vi "ChannelSounder.vi"() -> ()   [LabVIEW 2018]
uses:
  <instrlib>/niUSRP/niUSRP Fetch Rx Data (CDB WDT).vi
  <vilib>/measure/maspectr.llb/FFT Power Spectrum and PSD for 1 Chan (CDB).vi
  <vilib>/measure/NI_MAPro.lvlib
panel:
  out "Acquired Signal":waveform(dbl)[](graph)
  out "Waveform Graph":cluster{"f0":dbl, "df":dbl, "magnitude":dbl[]}(graph)
  in  "number of samples":i64=100000
  in  "stop":bool
  out "error out":errorcluster
  out "coerced gain":dbl format="%#_6f"
  out "coerced carrier frequency":dbl=100000.0 format="%#_6p"
  out "coerced IQ rate":dbl=100000.0 format="%#_6p"
  in  "active antenna":string="RX2"
  in  "carrier frequency":dbl=867999999.0 format="%#_6p"
  in  "IQ rate":dbl=100000.0 format="%#_6p"
  in  "Rx gain [dB]":dbl format="%#_6f"
  in  "device IP":refnum<k15>="192.168.10.2"
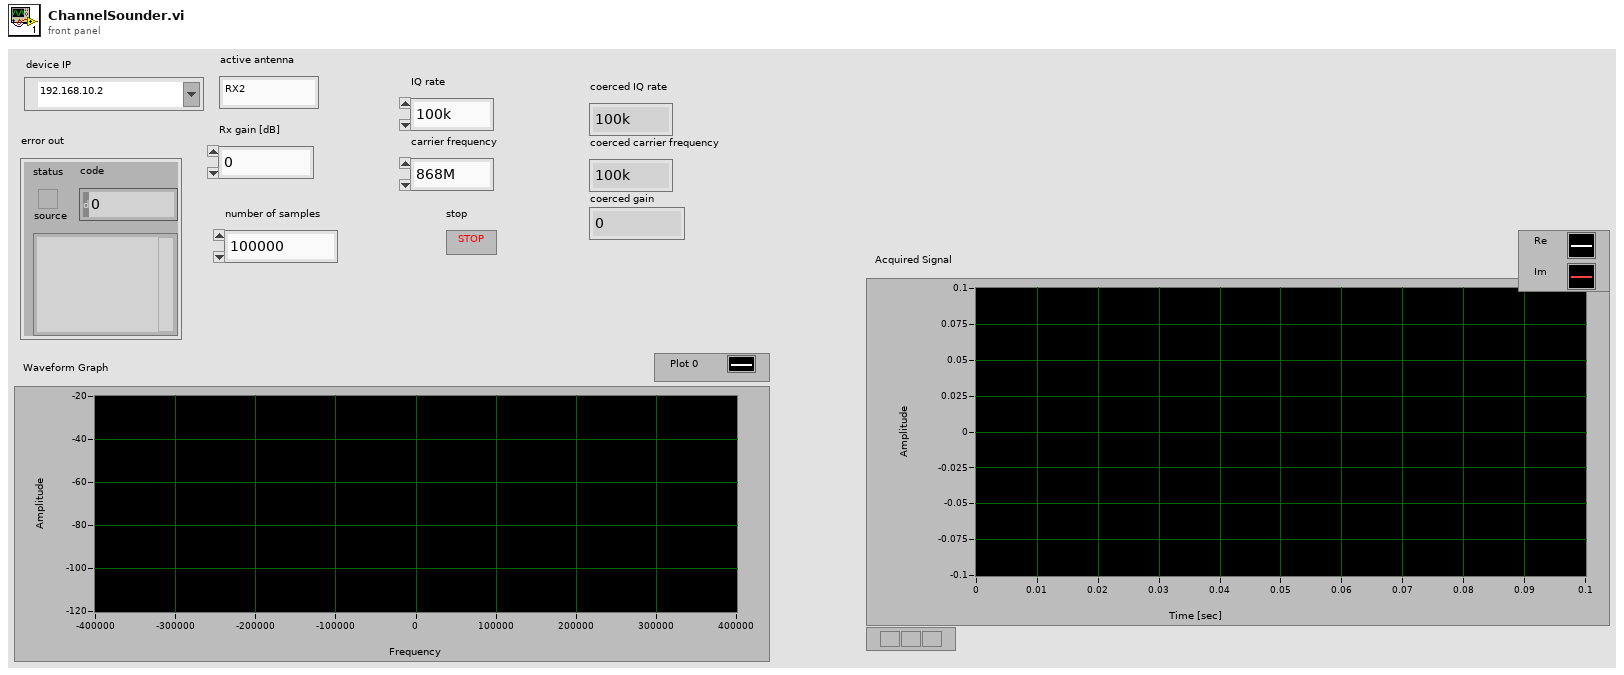
[diagram p1: front panel]
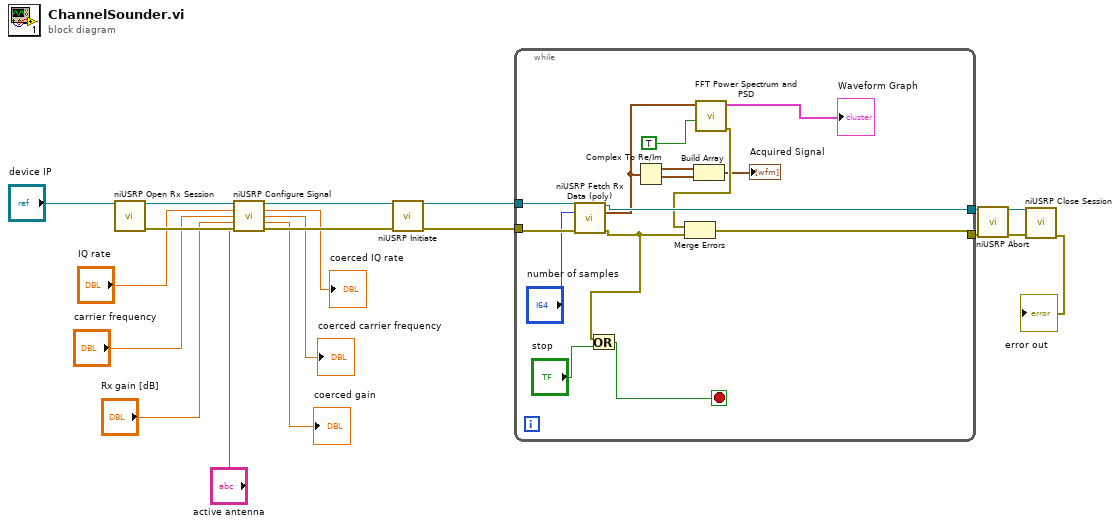
[diagram p0: block diagram]
diagram:
  n1 = call <instrlib>:"niUSRP Open Rx Session.vi"("device names"="device IP") -> ("session handle out"=w19:refnum<k15>, "error out"=w18:errorcluster)  [unwired: 13 in]
  n2 = call <instrlib>:"niUSRP Configure Signal.vi"("session handle"=w19, "IQ rate"="IQ rate", "carrier frequency"="carrier frequency", "gain"="Rx gain [dB]", "error in (no error)"=w18, "active antenna"="active antenna") -> ("session handle out"=w17:refnum<k15>, "coerced IQ rate"=→"coerced IQ rate":dbl, "coerced carrier frequency"=→"coerced carrier frequency":dbl, "coerced gain"=→"coerced gain":dbl, "error out"=w16:errorcluster)  [unwired: 5 in]
  n3 = call <instrlib>:"niUSRP Initiate.vi"("session handle"=w17, "error in (no error)"=w16) -> ("session handle out"=w6:refnum<k15>, "error out"=w7:errorcluster)  [unwired: 12 in]
  n4 = while {
    tunnel: w7 -> [w33]
    tunnel: w6 -> [w34]
    tunnel: [w31] -> w5
    tunnel: [w28] -> w4
    stop <- w32 stop-if-true
    n5 = call-poly <instrlib>:"niUSRP Fetch Rx Data (poly).vi"("session handle"=w34, "number of samples"="number of samples", "error in (no error)"=w33) -> ("session handle out"=w31:refnum<k15>, "data"=w20:waveform(cdb), "error out"=w26:errorcluster)  [unwired: 9 in, 1 out]
    n6 = Or(x=w26, y="stop") -> (x .or. y?=w32:bool)
    n7 = Complex To Re/Im(x + iy=w20) -> (x=w23:waveform(dbl), y=w22:waveform(dbl))
    n8 = Build Array(w23, w22) -> (→"Acquired Signal":waveform(dbl)[])
    n9 = call-poly <vilib>:"FFT Power Spectrum and PSD.vi"("dB On (F)"=TRUE, "time signal"=w20) -> ("error out"=w27:errorcluster, "Power Spectrum / PSD"=→"Waveform Graph":cluster{"f0":dbl, "df":dbl, "magnitude":dbl[]})  [unwired: 6 in, 2 out]
    n10 = Merge Errors(w27, w26) -> (w28:errorcluster)
  }
  n11 = call <instrlib>:"niUSRP Abort.vi"("session handle"=w5, "error in (no error)"=w4) -> ("session handle out"=w3:refnum<k15>, "error out"=w2:errorcluster)  [unwired: 12 in]
  n12 = call <instrlib>:"niUSRP Close Session.vi"("session handle"=w3, "error in (no error)"=w2) -> ("error out"=→"error out":errorcluster)  [unwired: 13 in]
